vi "Matrix_ElementSum.vi"(11 "input matrix":T1) -> (3 "Sum":dbl)   [LabVIEW 2019, in "Trajectory_Library.lvlib"]
doc: "Creates a new LINEAR SYSTEM data cluster with the specified values. \n\n\nInputs: \n - XXX -- XXX.\n\nOutputs:\n - XXX -- XXX."
uses:
  <vilib>/Analysis/Matrix/Datatypes/RealMatrix.ctl
  Trajectory_Library.lvlib
  <vilib>/Analysis/Matrix/NI_Matrix.lvlib
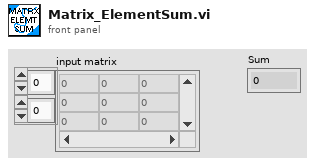
[diagram p1: front panel]
types:
  T1 = typedef "NI_Matrix.lvlib/RealMatrix.ctl" = dbl[][]
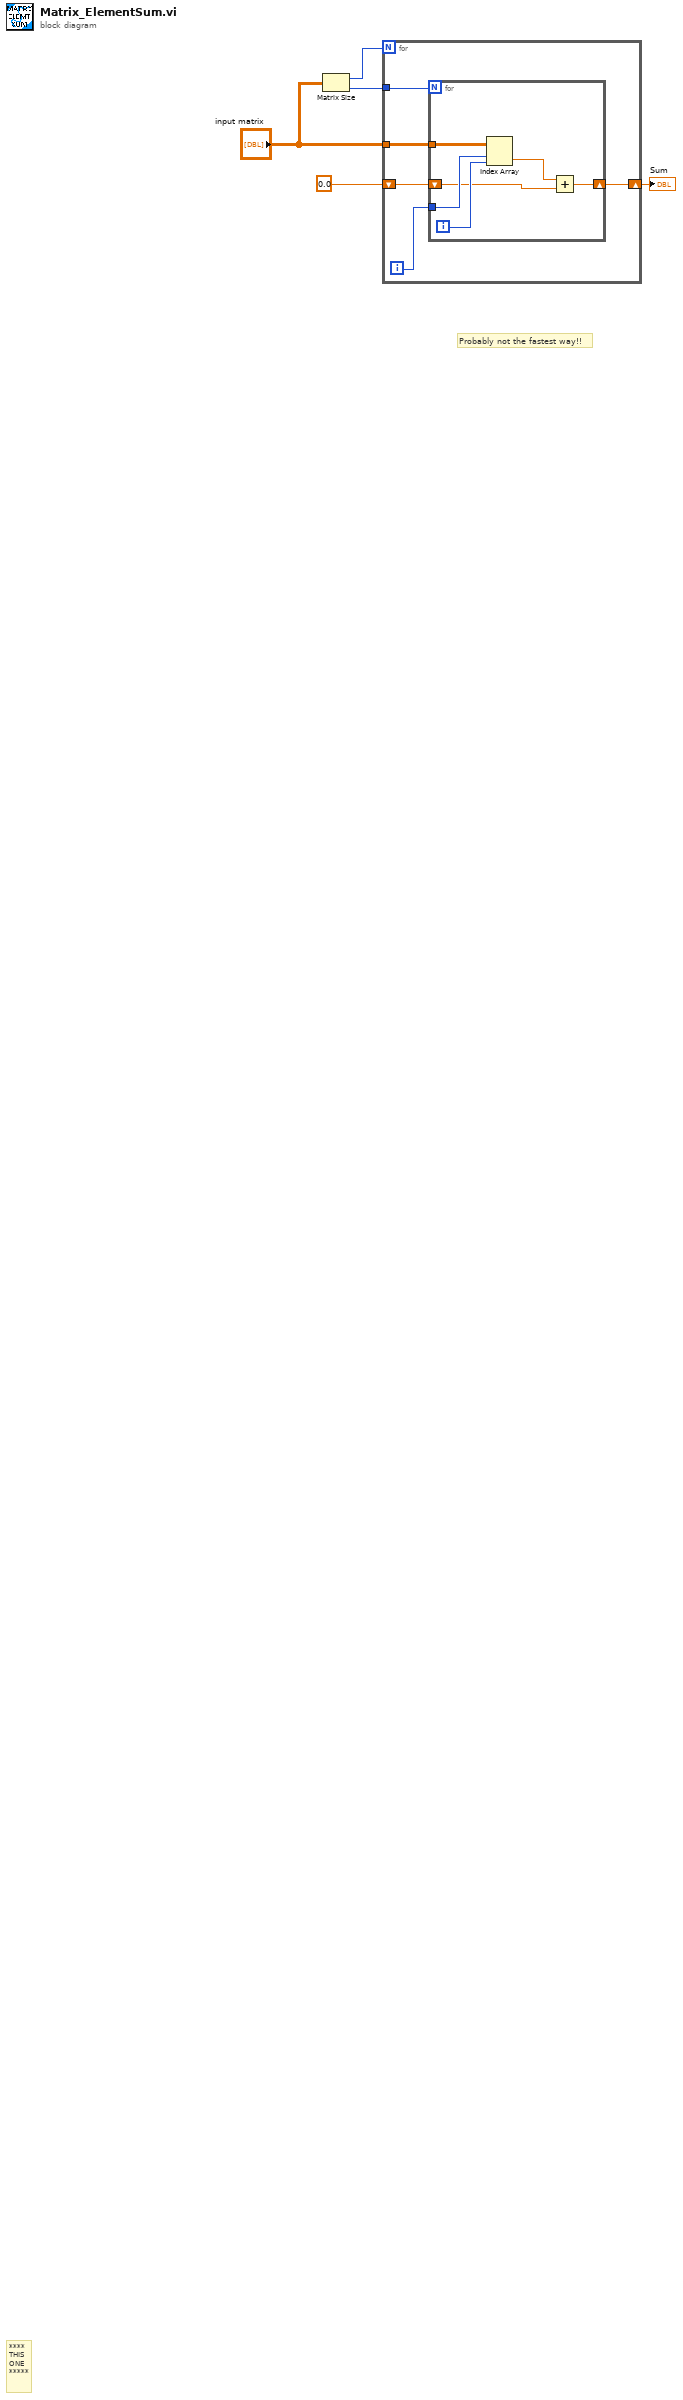
[diagram p0: block diagram]
diagram:
  # "Probably not the fastest way!!"
  # "****\nTHIS\nONE\n*****"
  n1 = Matrix Size(0:"input matrix") -> (1:w4:i32, 2:w3:i32)
  n2 = for {
    N: w4 -> [_]
    tunnel: w3 -> [w8]
    shift-right: [w6] -> w1
    shift-left: 0.0 -> [w7]
    tunnel: "input matrix" -> [w10]
    i -> [w9]
    n3 = for {
      N: w8 -> [_]
      tunnel: w9 -> [w15]
      shift-right: [w13] -> w6
      shift-left: w7 -> [w11]
      tunnel: w10 -> [w16]
      i -> [w14]
      n4 = Index Array(array=w16, index (row)=w15, index (col)=w14) -> (element=w12:dbl)
      n5 = Add(x=w12, y=w11) -> (x+y=w13:dbl)
    }
  }
  "Sum" <- w1
